vi "Location.Vertical.Update.vi"(10 "Vertical Change":i16, 11 "location in":T1) -> (3 "location out":T1)   [LabVIEW 2019, in "Structures.lvclass"]
uses:
  Structures.lvclass
  <vilib>/Utility/miscctls.llb/LVPointTypeDef.ctl
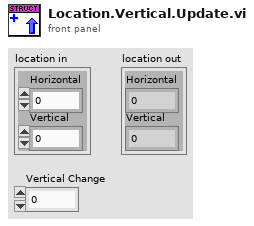
[diagram p1: front panel]
types:
  T1 = typedef "LVPointTypeDef.ctl" = cluster{"Horizontal":i16, "Vertical":i16}
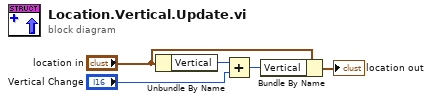
[diagram p0: block diagram]
diagram:
  n1 = Unbundle By Name("location in") -> ("Vertical"=w1:i16)
  n2 = Add(x=w1, y="Vertical Change") -> (x+y=w3:i16)
  n3 = Bundle By Name(cluster="location in", "Vertical"=w3) -> (→"location out":T1)
